vi "Square.vi"(0 "error in":errorcluster, 5 "Amount of Points":i32, 7 "Amplitude":dbl, 9 "Duty Cycle":dbl=0.01 min=0.01 max=0.99, 11 "DC Offset":dbl) -> (4 "error IO":errorcluster, 6 "Square Wave Array":dbl[](array[numeric]))   [LabVIEW 2020]
panel:
  out "Waveform Graph":dbl[](graph)
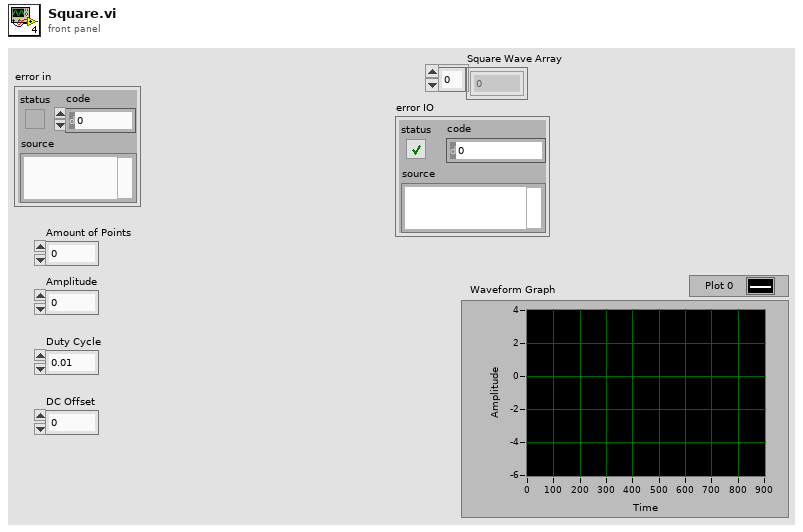
[diagram p1: front panel]
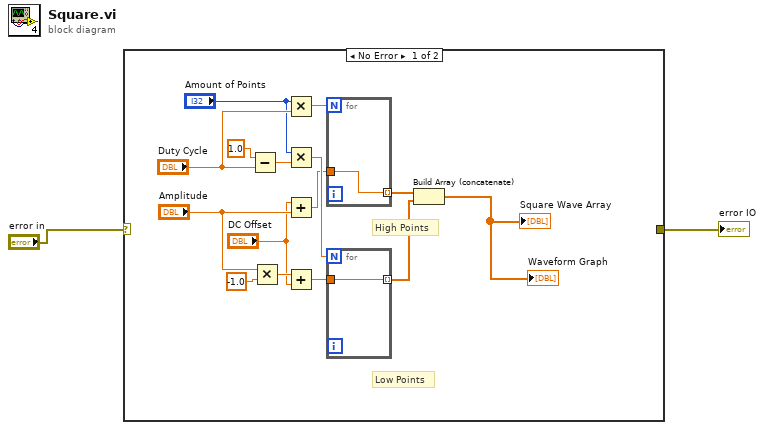
[diagram p0: block diagram]
diagram:
  n1 = case shown="No Error" "error in" {
    selector: "error in" -> [_ w20]
    tunnel: [_ w20] -> w1
    frame No Error {
      # "Low Points"
      # "High Points"
      n2 = Subtract(x=1.0, y="Duty Cycle") -> (x-y=w14:dbl)
      n3 = Multiply(x="Amplitude", y=-1.0) -> (x*y=w10:dbl)
      n4 = Multiply(x="Amount of Points", y="Duty Cycle") -> (x*y=w17:dbl)
      n5 = Multiply(x="Amount of Points", y=w14) -> (x*y=w13:dbl)
      n6 = Add(x="DC Offset", y="Amplitude") -> (x+y=w5:dbl)
      n7 = Add(x=w10, y="DC Offset") -> (x+y=w6:dbl)
      n8 = for {
        N: w17 -> [_]
        tunnel: w5 -> [w19]
        tunnel: [w19] -> w9 mode=indexing
      }
      n9 = for {
        N: w13 -> [_]
        tunnel: w6 -> [w18]
        tunnel: [w18] -> w8 mode=indexing
      }
      n10 = Build Array (concatenate)(w9, w8) -> (→"Waveform Graph" →"Square Wave Array":dbl[])
    }
    frame Error {
    }
  }
  "error IO" <- w1
